vi "Initialize.vi"(8 "error in (no error)":errorcluster, 11 "Test Manager in":refnum<class "Basic Test Manager.lvclass">) -> (0 "error out":errorcluster, 3 "Test Manager out":refnum<class "Basic Test Manager.lvclass">)   [LabVIEW 2013, in "Caraya.lvlib" / "Basic Test Manager.lvclass"]
uses:
  Basic Test Manager.lvclass
  Basic Test Manager.lvclass/Basic Test Manager.ctl
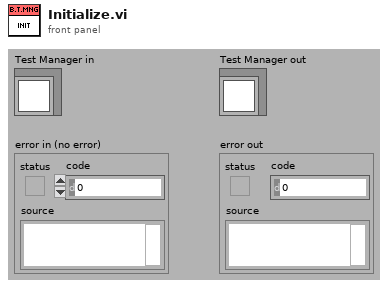
[diagram p1: front panel]
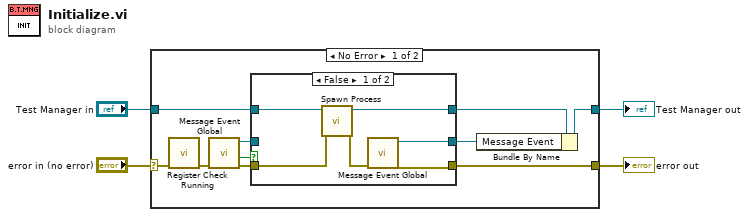
[diagram p0: block diagram]
diagram:
  n1 = case shown="No Error" "error in (no error)" {
    selector: "error in (no error)" -> [w11 w25]
    tunnel: [w13 w25] -> w2
    tunnel: [w8 w24] -> w4
    tunnel: "Test Manager in" -> [w14 w24]
    frame No Error {
      n2 = call "Register Check Running.vi"("error in (no error)"=w11) -> ("error out"=w6:errorcluster)  [unwired: 9 in, 1 out]
      n3 = call "Message Event Global.vi"("error in (no error)"=w6) -> ("error out"=w5:errorcluster, "Is Set?"=w7:bool, "Message Event out"=w9:refnum<user-event>)  [unwired: 7 in, 1 out]
      n4 = case shown="False" w7 {
        tunnel: w5 -> [w15 w21]
        tunnel: w14 -> [w20 w23]
        tunnel: [w19 w23] -> w12
        tunnel: [w16 w21] -> w13
        tunnel: [w18 w22] -> w10
        tunnel: w9 -> [_ w22]
        frame False {
          n5 = call "Spawn Process.vi"("error in (no error)"=w15, "Test Manager in"=w20) -> ("error out"=w17:errorcluster, "Test Manager out"=w19:refnum<class "Basic Test Manager.lvclass">)  [unwired: 8 in]
          n6 = call "Message Event Global.vi"("error in (no error)"=w17) -> ("error out"=w16:errorcluster, "Message Event out"=w18:refnum<user-event>)  [unwired: 7 in, 2 out]
        }
        frame True {
        }
      }
      n7 = Bundle By Name(cluster=w12, "Message Event"=w10) -> (w8:refnum<class "Basic Test Manager.lvclass">)
    }
    frame Error {
    }
  }
  "Test Manager out" <- w4
  "error out" <- w2
